vi "Driver - DTACQ - Open TCP Connection.vi"(8 "error in":errorcluster, 11 "DTACQ Connection Data In":T1={"Description"="", "Address"="", "Port"=0, "timeout (ms)"=5000, "Termination Character"="\n", "TCP Connection Reference"=refnum, "Open Connection"=FALSE}) -> (0 "error out":errorcluster, 3 "DTACQ Connection Data Out":T1={"Description"="", "Address"="", "Port"=0, "timeout (ms)"=5000, "Termination Character"="\n", "TCP Connection Reference"=refnum, "Open Connection"=FALSE})   [LabVIEW 2017, in "Communications Library.lvlib"]
doc: "Opens a TCP connection to the specified IP address and port, if one is not already open.\n\nIf the connection is already open, does nothing."
uses:
  Communications Library.lvlib
  Typedefs/DTACQ Connection Data--Cluster.ctl
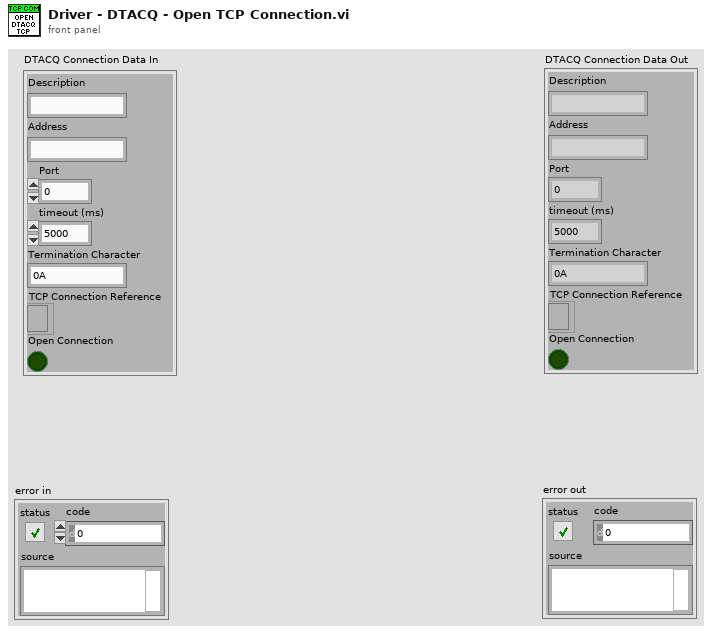
[diagram p1: front panel]
types:
  T1 = typedef "Communications Library.lvlib/DTACQ Connection Data--Cluster.ctl" = cluster{"Description":string, "Address":string, "Port":u16, "timeout (ms)":i32, "Termination Character":string, "TCP Connection Reference":refnum<k5>, "Open Connection":bool}
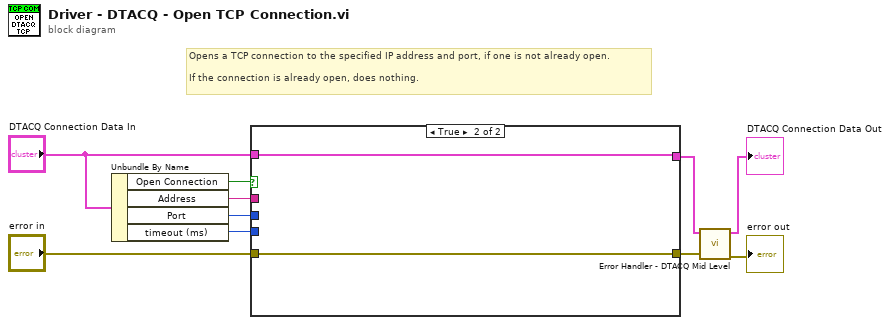
[diagram p0: block diagram]
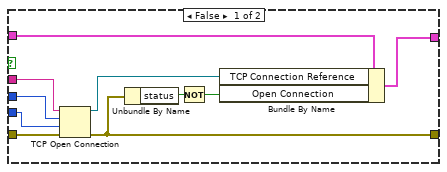
[diagram p2: hidden frame]
diagram:
  # "Opens a TCP connection to the specified IP address and port, if one is not already open.\n\nIf the connection is already open, does nothing."
  n1 = Unbundle By Name("DTACQ Connection Data In") -> ("Open Connection"=w9:bool, "Address"=w8:string, "Port"=w7:u16, "timeout (ms)"=w6:i32)
  n2 = case shown="True" w9 {
    tunnel: "error in" -> [w20 w21]
    tunnel: w8 -> [w19 _]
    tunnel: w7 -> [w18 _]
    tunnel: w6 -> [w17 _]
    tunnel: [w13 w21] -> w4
    tunnel: "DTACQ Connection Data In" -> [w16 w22]
    tunnel: [w14 w22] -> w3
    frame False {
      n3 = TCP Open Connection(address=w19, remote port or service name=w18, timeout ms (60000)=w17, error in (no error)=w20) -> (connection ID=w15:refnum<k5>, error out=w13:errorcluster)  [unwired: 1 in]
      n4 = Unbundle By Name(w13) -> ("status"=w12:bool)
      n5 = Not(x=w12) -> (.not. x?=w11:bool)
      n6 = Bundle By Name(cluster=w16, "TCP Connection Reference"=w15, "Open Connection"=w11) -> (w14:T1)
    }
    frame True {
    }
  }
  n7 = call "Error Handler - DTACQ Mid Level.vi"("error in"=w4, "DTACQ Connection Data In"=w3) -> ("error out"=→"error out":errorcluster, "DTACQ Connection Data Out"=→"DTACQ Connection Data Out":T1)  [unwired: 7 in, 1 out]
